vi "GlobeVaribles.vi"() -> ()   [LabVIEW 2016]
panel:
  in  "CFilePath":string
  in  "SFilePath":string
  out "Sample?":bool
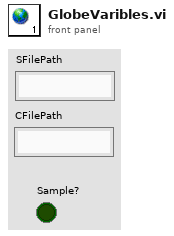
[diagram p1: front panel]
diagram:
